vi "sendProtocol.vi"(8 "error in (no error)":errorcluster, 9 "GoTo position":dbl, 10 "command":string, 11 "TCP Network Connection in":refnum<k5>) -> (0 "error out":errorcluster, 3 "TCP Network Connection out":refnum<k5>)   [LabVIEW 2019, in "ESP301viaTCPIP.lvlib"]
uses:
  ESP301viaTCPIP.lvlib
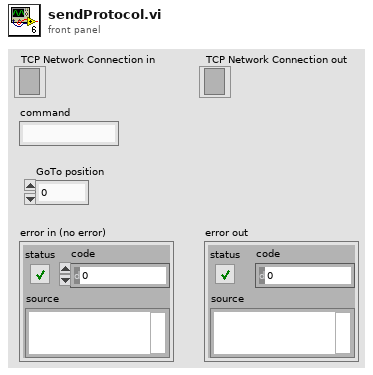
[diagram p1: front panel]
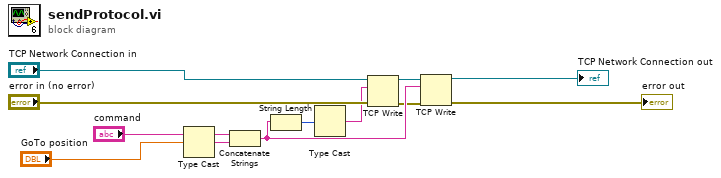
[diagram p0: block diagram]
diagram:
  n1 = Type Cast(x="GoTo position") -> (*(type *) &x=w5:string)  [unwired: 1 in]
  n2 = Concatenate Strings("command", w5) -> (w6:string)
  n3 = String Length(string=w6) -> (length=w3:i32)
  n4 = Type Cast(x=w3) -> (*(type *) &x=w4:string)  [unwired: 1 in]
  n5 = TCP Write(connection ID="TCP Network Connection in", data in=w4, error in (no error)="error in (no error)") -> (connection ID out=w1:refnum<k5>, error out=w2:errorcluster)  [unwired: 1 in, 1 out]
  n6 = TCP Write(connection ID=w1, data in=w6, error in (no error)=w2) -> (connection ID out=→"TCP Network Connection out":refnum<k5>, error out=→"error out":errorcluster)  [unwired: 1 in, 1 out]
